vi "ChessTopVI.vi"() -> ()   [LabVIEW 2014]
panel:
  out "Whose Turn":string
  out "Draw":bool
  out "Black:":string
  out "Target Piece":i32
  out "Selected Piece":i32
  out "White:":string
  out "LastMovePiece":cluster{"Row":i32, "Column":i32, "IsMove":bool}
  out "AttachablePositionIndexes":i32[](array[numeric])
  out "AttachablePosition":bool[][](array[boolean])
  out "Target Piece Index":i32
  out "Selected Piece Index":i32
  in  "stop":bool
  out "Board":i32[][](array[numeric])=[[-3, -5, -4, -2, -1, -4, -5, -3], [-6, -6, -6, -6, -6, -6, -6, -6], [0, 0, 0, 0, 0, 0, 0, 0], [0, 0, 0, 0, 0, 0, 0, 0], [0, 0, 0, 0, 0, 0, 0, 0], [0, 0, 0, 0, 0, 0, 0, 0], [6, 6, 6, 6, 6, 6, 6, 6], [3, 5, 4, 2, 1, 4, 5, 3]]
  out "Black/White Turn (T/F)":bool
  out "Castling State":bool[][](array[boolean])
  in  "Cluster":T1
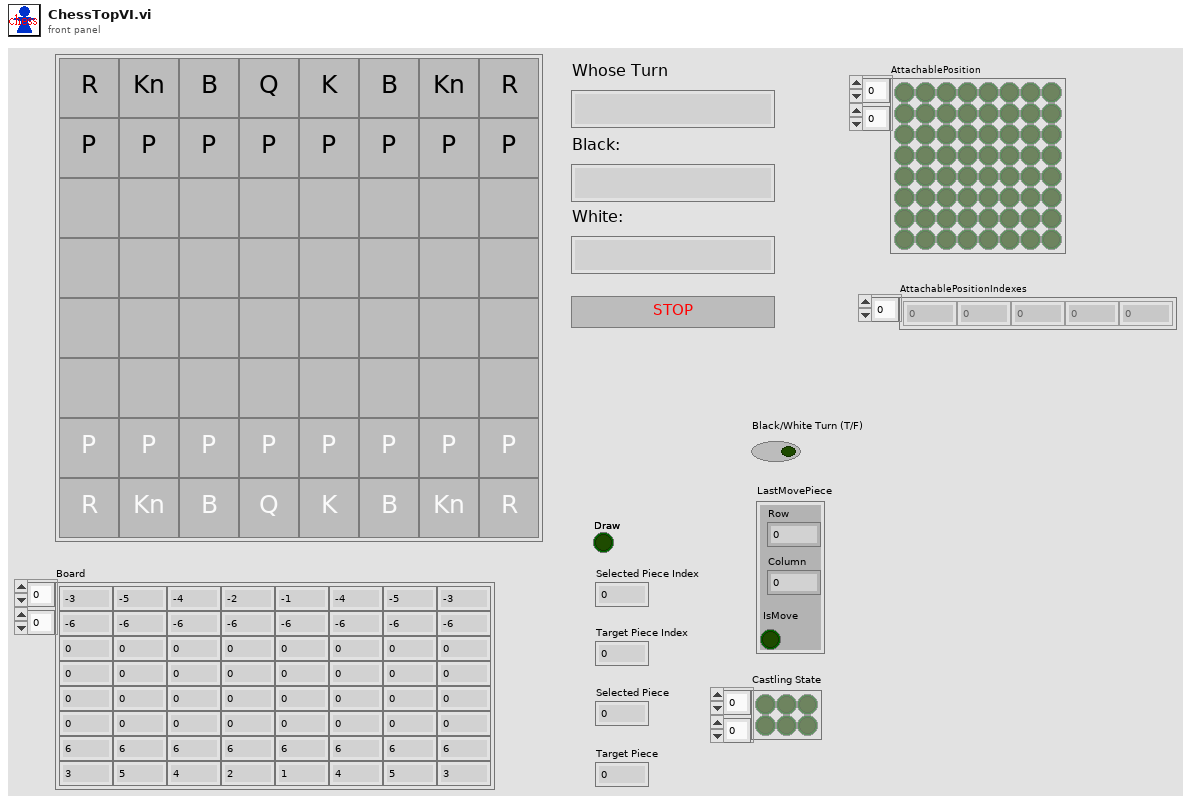
[diagram p1: front panel]
types:
  T1 = cluster{"OK Button":bool, "OK Button 2":bool, "OK Button 3":bool, "OK Button 4":bool, "OK Button 5":bool, "OK Button 6":bool, "OK Button 3":bool, "OK Button 7":bool, "OK Button 8":bool, "OK Button 9":bool, "OK Button 10":bool, "OK Button 11":bool, "OK Button 12":bool, "OK Button 13":bool, "OK Button 14":bool, "OK Button 15":bool, "OK Button 16":bool, "OK Button 17":bool, "OK Button 18":bool, "OK Button 19":bool, "OK Button 20":bool, "OK Button 21":bool, "OK Button 22":bool, "OK Button 23":bool, "OK Button 24":bool, "OK Button 25":bool, "OK Button 26":bool, "OK Button 27":bool, "OK Button 28":bool, "OK Button 29":bool, "OK Button 30":bool, "OK Button 31":bool, "OK Button 32":bool, "OK Button 33":bool, "OK Button 34":bool, "OK Button 35":bool, "OK Button 36":bool, "OK Button 37":bool, "OK Button 38":bool, "OK Button 39":bool, "OK Button 40":bool, "OK Button 41":bool, "OK Button 42":bool, "OK Button 43":bool, "OK Button 44":bool, "OK Button 45":bool, "OK Button 46":bool, "OK Button 47":bool, "OK Button 48":bool, "OK Button 49":bool, "OK Button 50":bool, "OK Button 51":bool, "OK Button 52":bool, "OK Button 53":bool, "OK Button 54":bool, "OK Button 55":bool, "OK Button 56":bool, "OK Button 57":bool, "OK Button 58":bool, "OK Button 59":bool, "OK Button 60":bool, "OK Button 61":bool, "OK Button 62":bool, "OK Button 63":bool}
  T2 = enum16{"init", "wait", "selected", "move/attack", "promotion", "checkmate"}
  T3 = cluster{"[0]":bool, "[1]":bool, "[2]":bool, "[3]":bool, "[4]":bool, "[5]":bool, "[6]":bool, "[7]":bool, "[8]":bool, "[9]":bool, "[10]":bool, "[11]":bool, "[12]":bool, "[13]":bool, "[14]":bool, "[15]":bool, "[16]":bool, "[17]":bool, "[18]":bool, "[19]":bool, "[20]":bool, "[21]":bool, "[22]":bool, "[23]":bool, "[24]":bool, "[25]":bool, "[26]":bool, "[27]":bool, "[28]":bool, "[29]":bool, "[30]":bool, "[31]":bool, "[32]":bool, "[33]":bool, "[34]":bool, "[35]":bool, "[36]":bool, "[37]":bool, "[38]":bool, "[39]":bool, "[40]":bool, "[41]":bool, "[42]":bool, "[43]":bool, "[44]":bool, "[45]":bool, "[46]":bool, "[47]":bool, "[48]":bool, "[49]":bool, "[50]":bool, "[51]":bool, "[52]":bool, "[53]":bool, "[54]":bool, "[55]":bool, "[56]":bool, "[57]":bool, "[58]":bool, "[59]":bool, "[60]":bool, "[61]":bool, "[62]":bool, "[63]":bool}
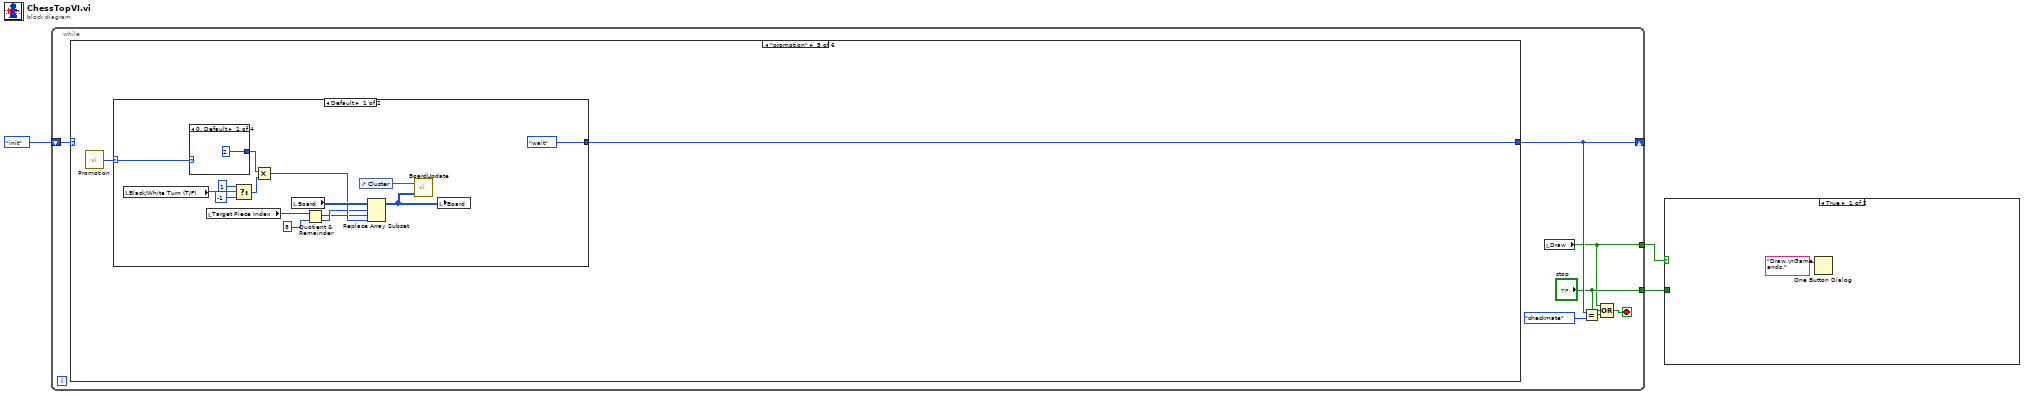
[diagram p0: block diagram]
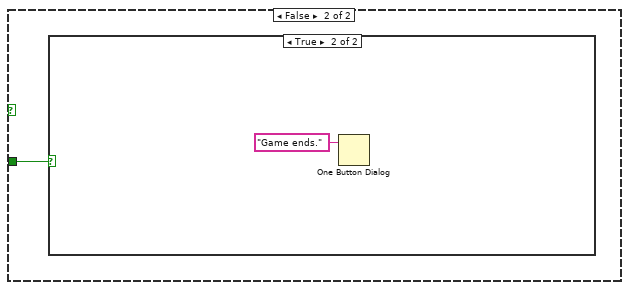
[diagram p2: hidden frame]
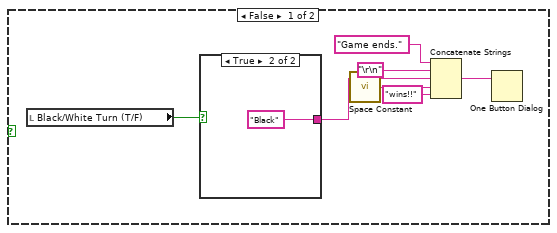
[diagram p3: hidden frame]
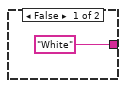
[diagram p4: hidden frame]
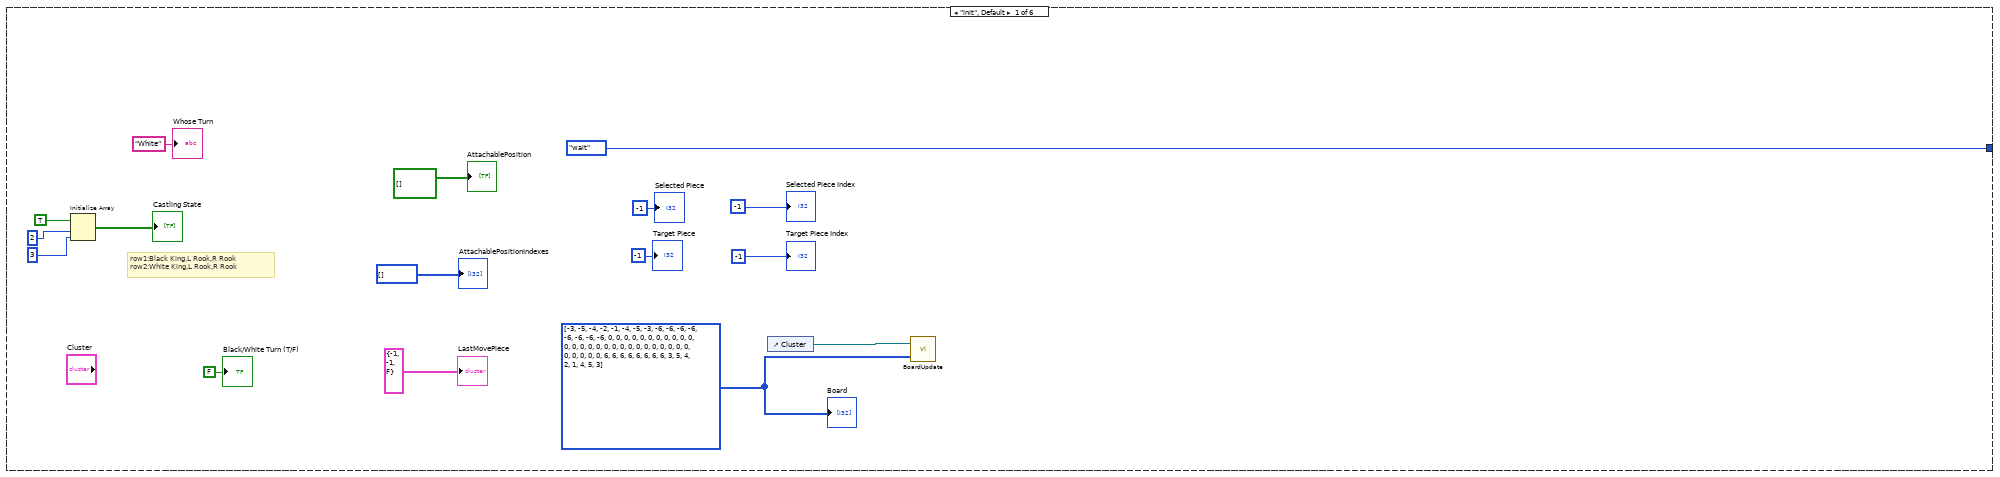
[diagram p5: hidden frame]
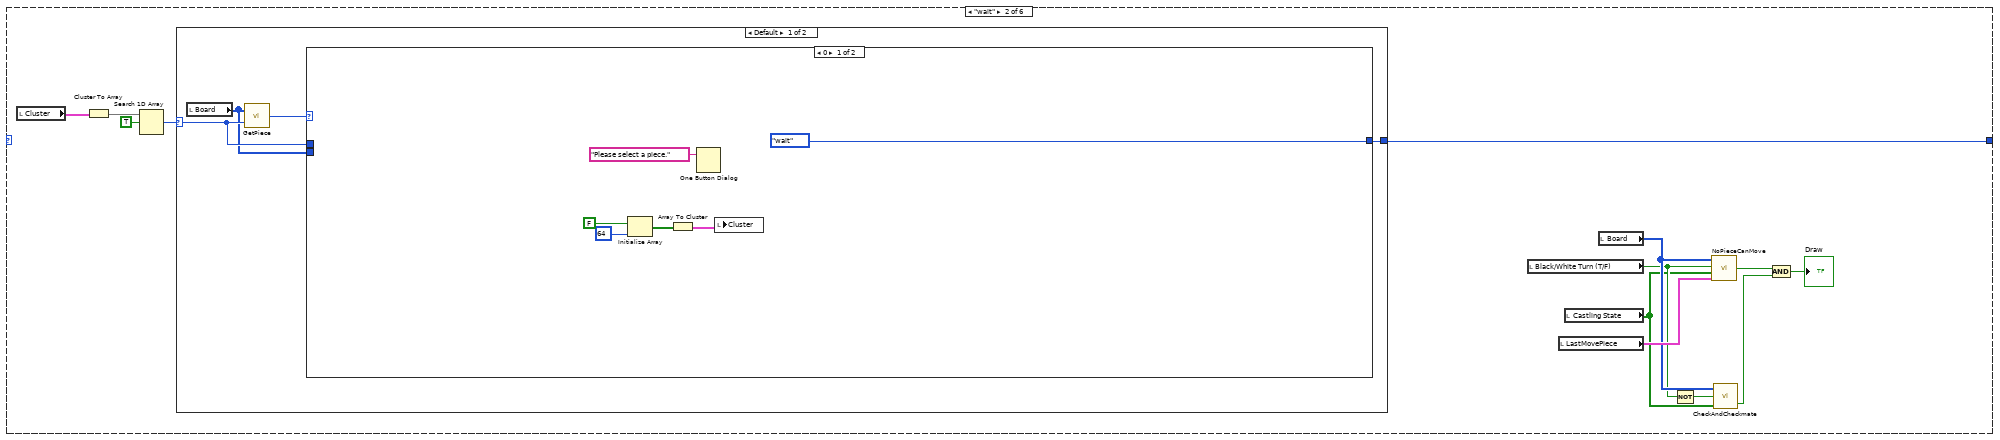
[diagram p6: hidden frame]
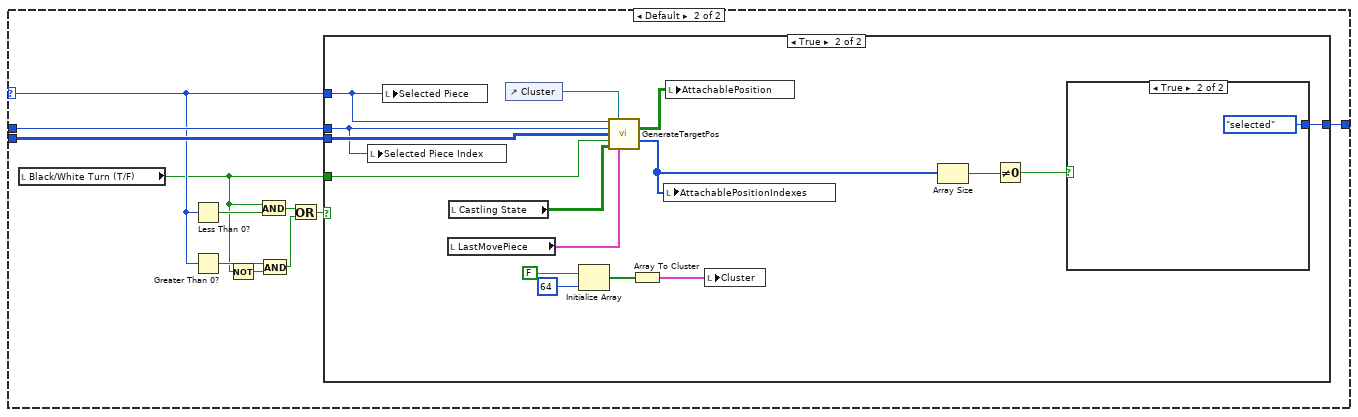
[diagram p7: hidden frame]
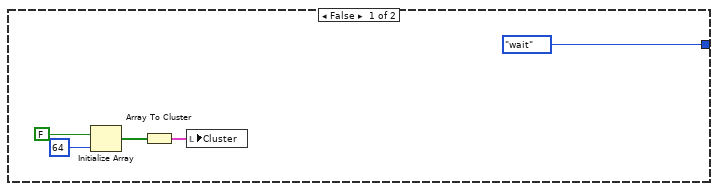
[diagram p8: hidden frame]
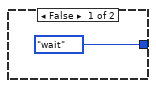
[diagram p9: hidden frame]
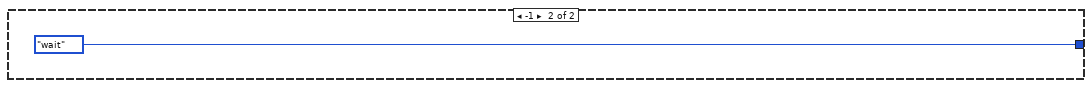
[diagram p10: hidden frame]
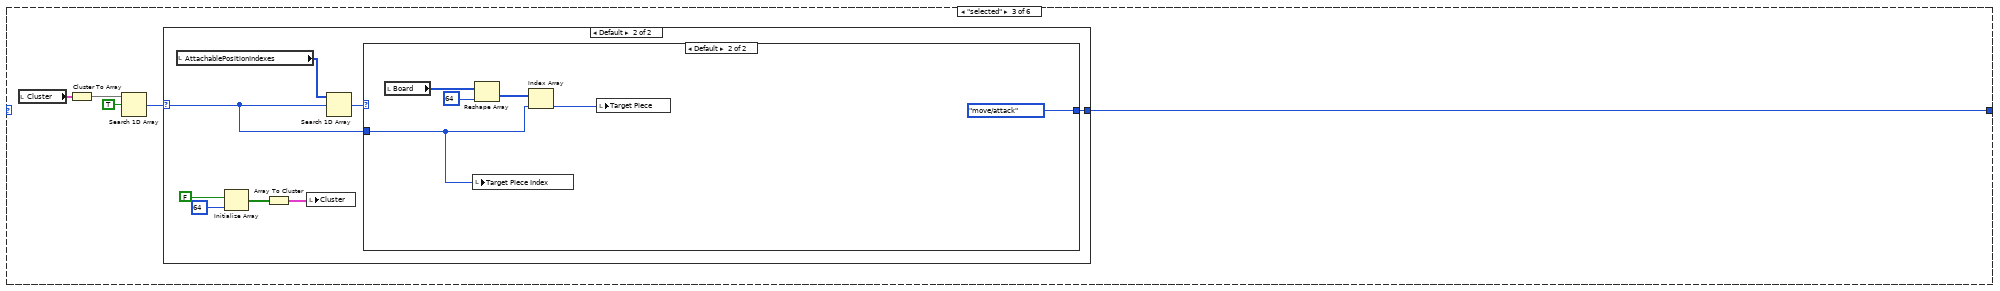
[diagram p11: hidden frame]
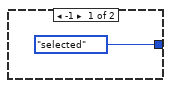
[diagram p12: hidden frame]
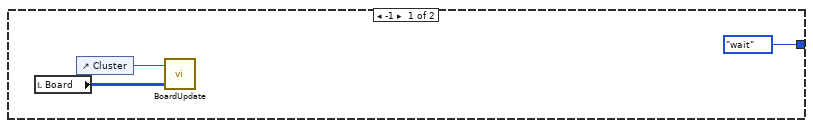
[diagram p13: hidden frame]
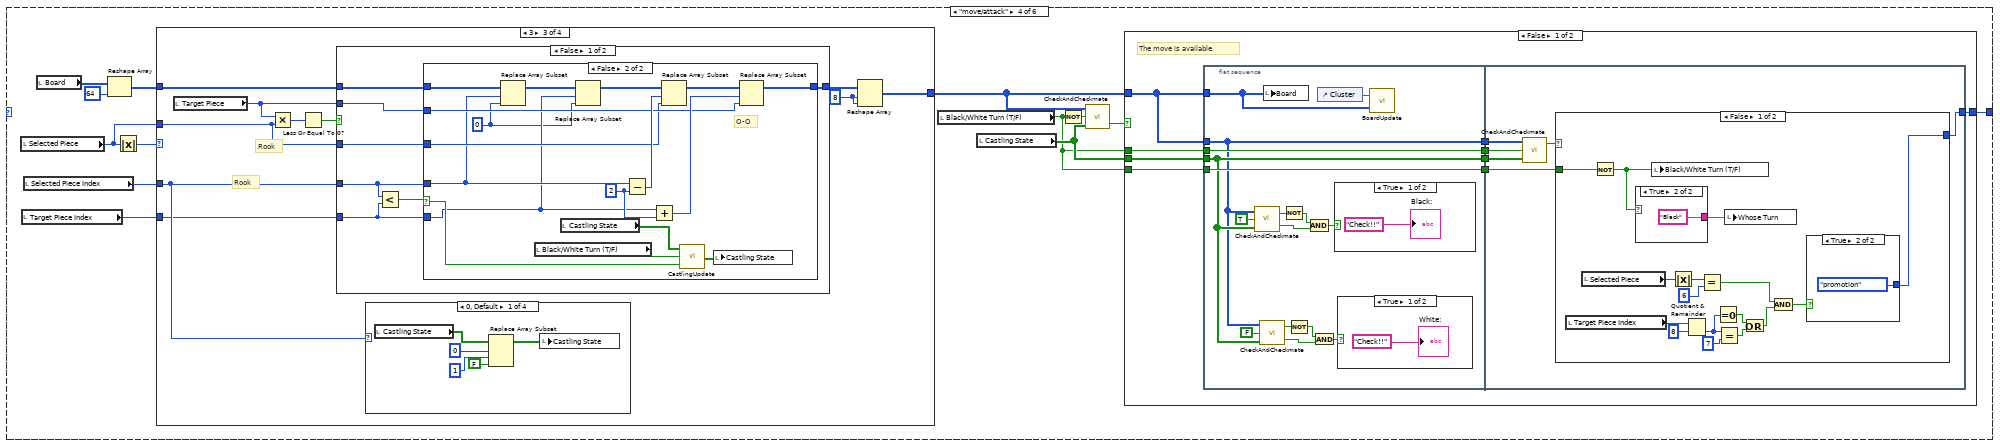
[diagram p14: hidden frame]
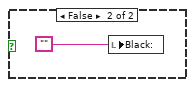
[diagram p15: hidden frame]
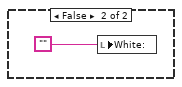
[diagram p16: hidden frame]
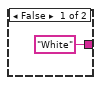
[diagram p17: hidden frame]
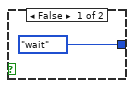
[diagram p18: hidden frame]
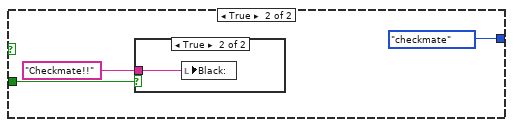
[diagram p19: hidden frame]
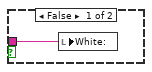
[diagram p20: hidden frame]
diagram:
  n1 = while {
    shift-right: [w8] -> _
    shift-left: T2."init" -> [w9]
    tunnel: ["stop"] -> w2
    tunnel: [w4] -> w1
    stop <- w6 stop-if-true
    n2 = case shown="\"promotion\"" w9 {
      tunnel: [T2."wait" w36 w89 w111 w412 T2."checkmate"] -> w8
      frame "init", Default {
        w12 = i32[][] [[-3, -5, -4, -2, -1, -4, -5, -3], [-6, -6, -6, -6, -6, -6, -6, -6], [0, 0, 0, 0, 0, 0, 0, 0], [0, 0, 0, 0, 0, 0, 0, 0], [0, 0, 0, 0, 0, 0, 0, 0], [0, 0, 0, 0, 0, 0, 0, 0], [6, 6, 6, 6, 6, 6, 6, 6], [3, 5, 4, 2, 1, 4, 5, 3]] ("Board")
        # "row1:Black King,L Rook,R Rook\nrow2:White King,L Rook,R Rook"
        n3 = Initialize Array(TRUE, 2, 3) -> (→"Castling State":bool[][])
        n4 = control-ref of="Cluster"() -> (w26:refnum<vi>)
        n5 = call "BoardUpdate.vi"("Array"=w12, "Clust Refnum"=w26) -> ()  [unwired: 1 in]
        "Black/White Turn (T/F)" <- FALSE ("Black/White Turn (T/F)")
        "Board" <- w12
        "LastMovePiece" <- cluster{"Row":i32, "Column":i32, "IsMove":bool} {"Row"=-1, "Column"=-1, "IsMove"=FALSE} ("LastMovePiece")
        "Selected Piece Index" <- -1 ("Selected Piece Index")
        "AttachablePosition" <- bool[][] [] ("AttachablePosition")
        "AttachablePositionIndexes" <- i32[] [] ("AttachablePositionIndexes")
        "Target Piece Index" <- -1 ("Target Index")
        "Selected Piece" <- -1 ("Selected Piece")
        "Target Piece" <- -1 ("Target Piece")
        "Whose Turn" <- "White" ("Whose Turn")
      }
      frame "wait" {
        n6 = local read "Cluster"() -> (w39:T1)
        n7 = Cluster To Array(cluster=w39) -> (array=w35:bool[])
        n8 = Search 1D Array(1D array=w35, element=TRUE) -> (index of element=w37:i32)  [unwired: 1 in]
        n9 = case shown="Default" w37 {
          selector: w37 -> [w41 _]
          tunnel: [w43 T2."wait"] -> w36
          frame Default {
            n10 = local read "Board"() -> (w40:i32[][])
            n11 = call "GetPiece.vi"("PieceIndex"=w41, "Board"=w40) -> ("Piece"=w42:i32)
            n12 = case shown="0" w42 {
              selector: w42 -> [_ w57]
              tunnel: [T2."wait" w60] -> w43
              tunnel: w41 -> [_ w58]
              tunnel: w40 -> [_ w59]
              frame 0 {
                n13 = Initialize Array(FALSE ("new element/subarray"), 64 ("dimension size")) -> (w47:bool[])
                n14 = Array To Cluster(array=w47) -> (cluster=w44:T3)
                n15 = One Button Dialog(message="Please select a piece.") -> ()  [unwired: 1 in, 1 out]
                n16 = local write "Cluster"(w44) -> ()
              }
              frame Default {
                n17 = local read "Black/White Turn (T/F)"() -> (w50:bool)
                n18 = Less Than 0?(x=w57) -> (x < 0?=w56:bool)
                n19 = Greater Than 0?(x=w57) -> (x > 0?=w53:bool)
                n20 = Not(x=w50) -> (.not. x?=w51:bool)
                n21 = And(x=w50, y=w56) -> (x .and. y?=w54:bool)
                n22 = And(x=w53, y=w51) -> (x .and. y?=w52:bool)
                n23 = Or(x=w54, y=w52) -> (x .or. y?=w55:bool)
                n24 = case shown="True" w55 {
                  tunnel: [T2."wait" w81] -> w60
                  tunnel: w59 -> [_ w78]
                  tunnel: w58 -> [_ w68]
                  tunnel: w57 -> [_ w67]
                  tunnel: w50 -> [_ w66]
                  frame False {
                    n25 = Initialize Array(FALSE ("new element/subarray"), 64 ("dimension size")) -> (w64:bool[])
                    n26 = Array To Cluster(array=w64) -> (cluster=w61:T3)
                    n27 = local write "Cluster"(w61) -> ()
                  }
                  frame True {
                    n28 = local write "Selected Piece Index"(w68) -> ()
                    n29 = local write "Selected Piece"(w67) -> ()
                    n30 = local read "LastMovePiece"() -> (w76:cluster{"Row":i32, "Column":i32, "IsMove":bool})
                    n31 = local read "Castling State"() -> (w77:bool[][])
                    n32 = control-ref of="Cluster"() -> (w79:refnum<vi>)
                    n33 = Initialize Array(FALSE ("new element/subarray"), 64 ("dimension size")) -> (w74:bool[])
                    n34 = call "GenerateTargetPos.vi"("Piece"=w67, "Clust Refnum"=w79, "Index"=w68, "Board"=w78, "Black/White Turn (T/F)"=w66, "Castling State"=w77, "LastMovePiece"=w76) -> ("AttachablePosition"=w80:bool[][], "AttachablePositionIndexes"=w71:i32[])  [unwired: 7 in]
                    n35 = Array To Cluster(array=w74) -> (cluster=w75:T3)
                    n36 = local write "AttachablePositionIndexes"(w71) -> ()
                    n37 = local write "AttachablePosition"(w80) -> ()
                    n38 = local write "Cluster"(w75) -> ()
                    n39 = Array Size(array=w71) -> (size(s)=w70:i32)
                    n40 = Not Equal To 0?(x=w70) -> (x != 0?=w69:bool)
                    n41 = case shown="True" w69 {
                      tunnel: [T2."wait" T2."selected"] -> w81
                      frame False {
                      }
                      frame True {
                      }
                    }
                  }
                }
              }
            }
          }
          frame -1 {
          }
        }
        n42 = local read "Black/White Turn (T/F)"() -> (w32:bool)
        n43 = local read "LastMovePiece"() -> (w34:cluster{"Row":i32, "Column":i32, "IsMove":bool})
        n44 = local read "Castling State"() -> (w31:bool[][])
        n45 = local read "Board"() -> (w33:i32[][])
        n46 = Not(x=w32) -> (.not. x?=w30:bool)
        n47 = call "NoPieceCanMove.vi"("LastMovePiece"=w34, "Castling State"=w31, "Black/White Turn (T/F)"=w32, "Board"=w33) -> ("NoPieceCanMove"=w28:bool)
        n48 = call "CheckAndCheckmate.vi"("Castling State"=w31, "Black/White Turn (T/F)"=w30, "Board"=w33) -> ("Check"=w29:bool)  [unwired: 1 out]
        n49 = And(x=w28, y=w29) -> (x .and. y?=→"Draw":bool)
      }
      frame "selected" {
        n50 = local read "Cluster"() -> (w86:T1)
        n51 = Cluster To Array(cluster=w86) -> (array=w87:bool[])
        n52 = Search 1D Array(1D array=w87, element=TRUE) -> (index of element=w85:i32)  [unwired: 1 in]
        n53 = case shown="Default" w85 {
          selector: w85 -> [_ w95]
          tunnel: [T2."selected" w98] -> w89
          frame -1 {
          }
          frame Default {
            n54 = local read "AttachablePositionIndexes"() -> (w97:i32[])
            n55 = Initialize Array(FALSE ("new element/subarray"), 64 ("dimension size")) -> (w91:bool[])
            n56 = Array To Cluster(array=w91) -> (cluster=w94:T3)
            n57 = local write "Cluster"(w94) -> ()
            n58 = Search 1D Array(1D array=w97, element=w95) -> (index of element=w96:i32)  [unwired: 1 in]
            n59 = case shown="Default" w96 {
              tunnel: [T2."wait" T2."move/attack"] -> w98
              tunnel: w95 -> [_ w103]
              frame -1 {
                n60 = local read "Board"() -> (w100:i32[][])
                n61 = control-ref of="Cluster"() -> (w99:refnum<vi>)
                n62 = call "BoardUpdate.vi"("Array"=w100, "Clust Refnum"=w99) -> ()  [unwired: 1 in]
              }
              frame Default {
                n63 = local read "Board"() -> (w106:i32[][])
                n64 = local write "Target Piece Index"(w103) -> ()
                n65 = Reshape Array(w106, 64 ("dimension size")) -> (w104:i32[])
                n66 = Index Array(array=w104, index=w103) -> (element=w102:i32)
                n67 = local write "Target Piece"(w102) -> ()
              }
            }
          }
        }
      }
      frame "move/attack" {
        n68 = local read "Selected Piece"() -> (w117:i32)
        n69 = local read "Target Piece Index"() -> (w118:i32)
        n70 = local read "Selected Piece Index"() -> (w119:i32)
        n71 = local read "Board"() -> (w115:i32[][])
        n72 = Reshape Array(w115, 64 ("dimension size")) -> (w114:i32[])
        n73 = Absolute Value(x=w117) -> (abs(x)=w120:i32)
        n74 = case shown="3" w120 {
          tunnel: w119 -> [w191 w200 w270 w349]
          tunnel: w118 -> [w186 w204 w269 w350]
          tunnel: w117 -> [w195 w198 w267 w347]
          tunnel: [w192 w202 w272 w346] -> w110
          tunnel: w114 -> [w190 w201 w274 w348]
          frame Default {
            w193 = 8 ("dimension size")
            n75 = Replace Array Subset(array=w190, new element=0 ("new element/subarray"), index=w191) -> (w196:i32[])
            n76 = Replace Array Subset(array=w196, new element=w195, index=w186) -> (w194:i32[])
            n77 = Reshape Array(w194, w193, w193) -> (w192:i32[][])
            n78 = Quotient & Remainder(x=w186, y=8) -> (x-y*floor(x/y)=w183:i32, floor(x/y)=w184:i32)
            n79 = local read "LastMovePiece"() -> (w188:cluster{"Row":i32, "Column":i32, "IsMove":bool})
            n80 = Bundle By Name(cluster=w188, "Row"=w184, "Column"=w183, "IsMove"=FALSE) -> (w187:cluster{"Row":i32, "Column":i32, "IsMove":bool})
            n81 = local write "LastMovePiece"(w187) -> ()
          }
          frame 1 {
            w205 = 8 ("dimension size")
            n82 = case shown="4, Default" w200 {
              frame 4, Default {
                n83 = local read "Castling State"() -> (w212:bool[][])
                n84 = Replace Array Subset(array=w212, new element=FALSE ("new element/subarray"), index (row)=0, index (col)=0 ("disabled index (col)")) -> (w208:bool[][])
                n85 = local write "Castling State"(w208) -> ()
              }
              frame 60 {
                n86 = local read "Castling State"() -> (w217:bool[][])
                n87 = Replace Array Subset(array=w217, new element=FALSE ("new element/subarray"), index (row)=1, index (col)=0 ("disabled index (col)")) -> (w213:bool[][])
                n88 = local write "Castling State"(w213) -> ()
              }
            }
            n89 = local read "Target Piece"() -> (w199:i32)
            n90 = Multiply(x=w199, y=w198) -> (x*y=w207:i32)
            n91 = Less Or Equal To 0?(x=w207) -> (x <= 0?=w206:bool)
            n92 = case shown="False" w206 {
              tunnel: w201 -> [w221 w264]
              tunnel: w200 -> [w222 w263]
              tunnel: w204 -> [w223 w262]
              tunnel: w198 -> [w219 w261]
              tunnel: [w220 w260] -> w203
              tunnel: w199 -> [w218 _]
              frame False {
                n93 = Greater?(x=w222, y=w223) -> (0:w224:bool)
                n94 = case shown="True" w224 {
                  selector: w224 -> [w232 w250]
                  tunnel: w223 -> [w226 w244]
                  tunnel: w222 -> [w227 w245]
                  tunnel: w221 -> [w240 w259]
                  tunnel: [w238 w257] -> w220
                  tunnel: w219 -> [w231 w249]
                  tunnel: w218 -> [w230 w248]
                  frame True {
                    w225 = 0
                    # "O-O-O"
                    n95 = Replace Array Subset(array=w240, new element=w225, index=w227) -> (w229:i32[])
                    n96 = local read "Black/White Turn (T/F)"() -> (w235:bool)
                    n97 = local read "Castling State"() -> (w234:bool[][])
                    n98 = Replace Array Subset(array=w229, new element=w225, index=w226) -> (w228:i32[])
                    n99 = Subtract(x=w227, y=2) -> (x-y=w237:i32)
                    n100 = Add(x=3, y=w226) -> (x+y=w236:i32)
                    n101 = call "CastlingUpdate.vi"("L/R (T/F)"=w232, "Black/White Turn (T/F)"=w235, "Castling State"=w234) -> ("Update Castling State"=w233:bool[][])
                    n102 = Replace Array Subset(array=w228, new element=w231, index=w237) -> (w239:i32[])
                    n103 = local write "Castling State"(w233) -> ()
                    n104 = Replace Array Subset(array=w239, new element=w230, index=w236) -> (w238:i32[])
                  }
                  frame False {
                    w243 = 0
                    w254 = 2 ("y")
                    # "O-O"
                    n105 = Replace Array Subset(array=w259, new element=w243, index=w245) -> (w247:i32[])
                    n106 = local read "Black/White Turn (T/F)"() -> (w253:bool)
                    n107 = local read "Castling State"() -> (w252:bool[][])
                    n108 = Replace Array Subset(array=w247, new element=w243, index=w244) -> (w246:i32[])
                    n109 = Add(x=w245, y=w254) -> (x+y=w256:i32)
                    n110 = Subtract(x=w244, y=w254) -> (x-y=w255:i32)
                    n111 = call "CastlingUpdate.vi"("L/R (T/F)"=w250, "Black/White Turn (T/F)"=w253, "Castling State"=w252) -> ("Update Castling State"=w251:bool[][])
                    n112 = Replace Array Subset(array=w246, new element=w249, index=w256) -> (w258:i32[])
                    n113 = local write "Castling State"(w251) -> ()
                    n114 = Replace Array Subset(array=w258, new element=w248, index=w255) -> (w257:i32[])
                  }
                }
              }
              frame True {
                # "attack/move"
                n115 = Replace Array Subset(array=w264, new element=0 ("new element/subarray"), index=w263) -> (w265:i32[])
                n116 = Replace Array Subset(array=w265, new element=w261, index=w262) -> (w260:i32[])
              }
            }
            n117 = Reshape Array(w203, w205, w205) -> (w202:i32[][])
          }
          frame 3 {
            w273 = 8 ("dimension size")
            # "Rook"
            # "Rook"
            n118 = local read "Target Piece"() -> (w268:i32)
            n119 = Multiply(x=w268, y=w267) -> (x*y=w276:i32)
            n120 = Less Or Equal To 0?(x=w276) -> (x <= 0?=w275:bool)
            n121 = case shown="False" w275 {
              tunnel: w274 -> [w282 w323]
              tunnel: [w283 w322] -> w271
              tunnel: w270 -> [w279 w321]
              tunnel: w269 -> [w280 w320]
              tunnel: w267 -> [w277 w319]
              tunnel: w268 -> [w278 _]
              frame False {
                n122 = Less?(x=w279, y=w280) -> (x < y?=w281:bool)
                n123 = case shown="False" w281 {
                  selector: w281 -> [w289 w310]
                  tunnel: w280 -> [w285 w303]
                  tunnel: w279 -> [w286 w304]
                  tunnel: w282 -> [w300 w318]
                  tunnel: [w298 w316] -> w283
                  tunnel: w277 -> [w293 w311]
                  tunnel: w278 -> [w294 w312]
                  frame True {
                    w284 = 0 ("Target Piece")
                    # "O-O-O"
                    n124 = Replace Array Subset(array=w300, new element=w284, index=w286) -> (w288:i32[])
                    n125 = local read "Black/White Turn (T/F)"() -> (w292:bool)
                    n126 = Replace Array Subset(array=w288, new element=w284, index=w285) -> (w287:i32[])
                    n127 = local read "Castling State"() -> (w291:bool[][])
                    n128 = Add(x=w286, y=3) -> (x+y=w297:i32)
                    n129 = Subtract(x=w285, y=2 ("x")) -> (x-y=w296:i32)
                    n130 = Replace Array Subset(array=w287, new element=w293, index=w297) -> (w299:i32[])
                    n131 = call "CastlingUpdate.vi"("L/R (T/F)"=w289, "Black/White Turn (T/F)"=w292, "Castling State"=w291) -> ("Update Castling State"=w290:bool[][])
                    n132 = local write "Castling State"(w290) -> ()
                    n133 = Replace Array Subset(array=w299, new element=w294, index=w296) -> (w298:i32[])
                  }
                  frame False {
                    w302 = 0 ("new element/subarray")
                    w313 = 2 ("y")
                    # "O-O"
                    n134 = Replace Array Subset(array=w318, new element=w302, index=w304) -> (w306:i32[])
                    n135 = local read "Black/White Turn (T/F)"() -> (w307:bool)
                    n136 = local read "Castling State"() -> (w308:bool[][])
                    n137 = Replace Array Subset(array=w306, new element=w302, index=w303) -> (w305:i32[])
                    n138 = Subtract(x=w304, y=w313) -> (x-y=w315:i32)
                    n139 = Add(x=w303, y=w313) -> (x+y=w314:i32)
                    n140 = Replace Array Subset(array=w305, new element=w311, index=w315) -> (w317:i32[])
                    n141 = call "CastlingUpdate.vi"("L/R (T/F)"=w310, "Black/White Turn (T/F)"=w307, "Castling State"=w308) -> ("Update Castling State"=w309:bool[][])
                    n142 = local write "Castling State"(w309) -> ()
                    n143 = Replace Array Subset(array=w317, new element=w312, index=w314) -> (w316:i32[])
                  }
                }
              }
              frame True {
                # "attack/move"
                n144 = Replace Array Subset(array=w323, new element=0 ("new element/subarray"), index=w321) -> (w324:i32[])
                n145 = Replace Array Subset(array=w324, new element=w319, index=w320) -> (w322:i32[])
              }
            }
            n146 = case shown="0, Default" w270 {
              frame 0, Default {
                n147 = local read "Castling State"() -> (w330:bool[][])
                n148 = Replace Array Subset(array=w330, new element=FALSE ("new element/subarray"), index (row)=0, index (col)=1 ("disabled index (col)")) -> (w326:bool[][])
                n149 = local write "Castling State"(w326) -> ()
              }
              frame 7 {
                n150 = local read "Castling State"() -> (w335:bool[][])
                n151 = Replace Array Subset(array=w335, new element=FALSE ("new element/subarray"), index (row)=0, index (col)=2 ("disabled index (col)")) -> (w331:bool[][])
                n152 = local write "Castling State"(w331) -> ()
              }
              frame 56 {
                n153 = local read "Castling State"() -> (w340:bool[][])
                n154 = Replace Array Subset(array=w340, new element=FALSE ("new element/subarray"), index (row)=1, index (col)=1 ("disabled index (col)")) -> (w336:bool[][])
                n155 = local write "Castling State"(w336) -> ()
              }
              frame 63 {
                n156 = local read "Castling State"() -> (w345:bool[][])
                n157 = Replace Array Subset(array=w345, new element=FALSE ("new element/subarray"), index (row)=1, index (col)=2 ("disabled index (col)")) -> (w341:bool[][])
                n158 = local write "Castling State"(w341) -> ()
              }
            }
            n159 = Reshape Array(w271, w273, w273) -> (w272:i32[][])
          }
          frame 6 {
            n160 = Subtract(x=w349, y=w350) -> (x-y=w352:i32)
            n161 = Absolute Value(x=w352) -> (abs(x)=w351:i32)
            n162 = case shown="Default" w351 {
              tunnel: w350 -> [w371 w398]
              tunnel: w349 -> [w372 w409]
              tunnel: w348 -> [w368 w410]
              tunnel: w347 -> [w360 w403]
              tunnel: [w365 w405] -> w346
              frame Default {
                w369 = 8 ("dimension size")
                w370 = 8
                # "attack: different column"
                n163 = local read "LastMovePiece"() -> (w356:cluster{"Row":i32, "Column":i32, "IsMove":bool})
                n164 = Quotient & Remainder(x=w372, y=w370) -> (x-y*floor(x/y)=w358:i32, floor(x/y)=w359:i32)
                n165 = Quotient & Remainder(x=w371, y=w370) -> (x-y*floor(x/y)=w362:i32, floor(x/y)=w361:i32)
                n166 = Reshape Array(w368, w369, w369) -> (w366:i32[][])
                n167 = Unbundle By Name(w356) -> ("Row"=w364:i32, "Column"=w363:i32, "IsMove"=w367:bool)
                n168 = case shown="False" w367 {
                  tunnel: w366 -> [w382 w395]
                  tunnel: [w380 w393] -> w365
                  tunnel: w364 -> [_ w392]
                  tunnel: w363 -> [_ w391]
                  tunnel: w362 -> [w375 w384]
                  tunnel: w361 -> [w374 w385]
                  tunnel: w360 -> [w379 w390]
                  tunnel: w359 -> [w377 w388]
                  tunnel: w358 -> [w378 w387]
                  tunnel: [w374 w385] -> w355
                  tunnel: [w375 w384] -> w354
                  tunnel: [FALSE FALSE] -> w353
                  frame False {
                    n169 = Replace Array Subset(array=w382, new element=0 ("new element/subarray"), index (row)=w377, index (col)=w378) -> (w381:i32[][])
                    n170 = Replace Array Subset(array=w381, new element=w379, index (row)=w374, index (col)=w375) -> (w380:i32[][])
                  }
                  frame True {
                    w386 = 0 ("new element/subarray")
                    # "En passant:吃過路兵"
                    n171 = Replace Array Subset(array=w395, new element=w386, index (row)=w388, index (col)=w387) -> (w389:i32[][])
                    n172 = Replace Array Subset(array=w389, new element=w386, index (row)=w392, index (col)=w391) -> (w394:i32[][])
                    n173 = Replace Array Subset(array=w394, new element=w390, index (row)=w385, index (col)=w384) -> (w393:i32[][])
                  }
                }
                n174 = Bundle By Name(cluster=w356, "Row"=w355, "Column"=w354, "IsMove"=w353) -> (w357:cluster{"Row":i32, "Column":i32, "IsMove":bool})
                n175 = local write "LastMovePiece"(w357) -> ()
              }
              frame 8, 16 {
                w404 = 8 ("dimension size")
                # "move: same column"
                n176 = Replace Array Subset(array=w410, new element=0 ("new element/subarray"), index=w409) -> (w407:i32[])
                n177 = Replace Array Subset(array=w407, new element=w403, index=w398) -> (w406:i32[])
                n178 = Quotient & Remainder(x=w398, y=8) -> (x-y*floor(x/y)=w399:i32, floor(x/y)=w400:i32)
                n179 = local read "LastMovePiece"() -> (w401:cluster{"Row":i32, "Column":i32, "IsMove":bool})
                n180 = Reshape Array(w406, w404, w404) -> (w405:i32[][])
                n181 = Bundle By Name(cluster=w401, "Row"=w400, "Column"=w399, "IsMove"=TRUE) -> (w402:cluster{"Row":i32, "Column":i32, "IsMove":bool})
                n182 = local write "LastMovePiece"(w402) -> ()
              }
            }
          }
        }
        n183 = local read "Black/White Turn (T/F)"() -> (w108:bool)
        n184 = local read "Castling State"() -> (w109:bool[][])
        n185 = Not(x=w108) -> (.not. x?=w113:bool)
        n186 = call "CheckAndCheckmate.vi"("Castling State"=w109, "Black/White Turn (T/F)"=w113, "Board"=w110) -> ("Check"=w112:bool)  [unwired: 1 out]
        n187 = case shown="False" w112 {
          tunnel: [w126 T2."selected"] -> w111
          tunnel: w110 -> [w121 _]
          tunnel: w108 -> [w129 _]
          tunnel: w109 -> [w128 _]
          tunnel: w108 -> [w127 _]
          frame False {
            # "The move is available."
            n188 = flat-sequence {
              tunnel: w121 -> [w130]
              tunnel: w127 -> [w144]
              tunnel: w128 -> [w131]
              tunnel: w129 -> [w145]
              tunnel: [w145] -> w125
              tunnel: [w131] -> w124
              tunnel: [w144] -> w123
              tunnel: [w130] -> w122
              tunnel: w121 -> [w142]
              tunnel: [w150] -> w126
              tunnel: w125 -> [w155]
              tunnel: w124 -> [w154]
              tunnel: w123 -> [w153]
              tunnel: w122 -> [w152]
              frame #0 {
                n189 = call "CheckAndCheckmate.vi"("Castling State"=w131, "Black/White Turn (T/F)"=TRUE, "Board"=w130) -> ("Check"=w135:bool, "Checkmate"=w137:bool)
                n190 = call "CheckAndCheckmate.vi"("Castling State"=w131, "Black/White Turn (T/F)"=FALSE, "Board"=w130) -> ("Check"=w138:bool, "Checkmate"=w141:bool)
                n191 = local write "Board"(w142) -> ()
                n192 = Not(x=w137) -> (.not. x?=w136:bool)
                n193 = Not(x=w141) -> (.not. x?=w139:bool)
                n194 = And(x=w136, y=w135) -> (x .and. y?=w134:bool)
                n195 = And(x=w139, y=w138) -> (x .and. y?=w140:bool)
                n196 = control-ref of="Cluster"() -> (w143:refnum<vi>)
                n197 = case shown="True" w134 {
                  frame True {
                    "Black:" <- "Check!!"
                  }
                  frame False {
                    n198 = local write "Black:"("") -> ()
                  }
                }
                n199 = case shown="True" w140 {
                  frame True {
                    "White:" <- "Check!!"
                  }
                  frame False {
                    n200 = local write "White:"("") -> ()
                  }
                }
                n201 = call "BoardUpdate.vi"("Array"=w142, "Clust Refnum"=w143) -> ()  [unwired: 1 in]
              }
              frame #1 {
                n202 = call "CheckAndCheckmate.vi"("Castling State"=w154, "Black/White Turn (T/F)"=w153, "Board"=w152) -> ("Checkmate"=w151:bool)  [unwired: 1 out]
                n203 = case shown="False" w151 {
                  tunnel: [w158 T2."checkmate"] -> w150
                  tunnel: w155 -> [w171 w176]
                  frame False {
                    n204 = local read "Target Piece Index"() -> (w167:i32)
                    n205 = local read "Selected Piece"() -> (w170:i32)
                    n206 = Not(x=w171) -> (.not. x?=w157:bool)
                    n207 = case shown="True" w157 {
                      tunnel: ["White" "Black"] -> w156
                      frame False {
                      }
                      frame True {
                      }
                    }
                    n208 = local write "Black/White Turn (T/F)"(w157) -> ()
                    n209 = Absolute Value(x=w170) -> (abs(x)=w169:i32)
                    n210 = Quotient & Remainder(x=w167, y=8) -> (floor(x/y)=w165:i32)  [unwired: 1 out]
                    n211 = Equal?(x=w169, y=6) -> (x = y?=w160:bool)
                    n212 = Equal To 0?(x=w165) -> (x = 0?=w162:bool)
                    n213 = Equal?(x=w165, y=7) -> (x = y?=w163:bool)
                    n214 = local write "Whose Turn"(w156) -> ()
                    n215 = Or(x=w162, y=w163) -> (x .or. y?=w161:bool)
                    n216 = And(x=w160, y=w161) -> (x .and. y?=w159:bool)
                    n217 = case shown="True" w159 {
                      tunnel: [T2."wait" T2."promotion"] -> w158
                      frame False {
                      }
                      frame True {
                      }
                    }
                  }
                  frame True {
                    n218 = case shown="True" w176 {
                      tunnel: "Checkmate!!" -> [w179 w180]
                      frame False {
                        n219 = local write "White:"(w179) -> ()
                      }
                      frame True {
                        n220 = local write "Black:"(w180) -> ()
                      }
                    }
                  }
                }
              }
            }
          }
          frame True {
            # "The move is not available."
            n221 = One Button Dialog(message="The move will make you be checked.") -> ()  [unwired: 1 in, 1 out]
          }
        }
      }
      frame "promotion" {
        n222 = call "Promotion.vi"() -> ("index of element"=w411:i32)  [unwired: 1 in]
        n223 = case shown="Default" w411 {
          selector: w411 -> [w427 _]
          tunnel: [T2."wait" T2."promotion"] -> w412
          frame Default {
            n224 = local read "Black/White Turn (T/F)"() -> (w414:bool)
            n225 = case shown="0, Default" w427 {
              tunnel: [2 3 4 5] -> w422
              frame 0, Default {
              }
              frame 1 {
              }
              frame 2 {
              }
              frame 3 {
              }
            }
            n226 = local read "Target Piece Index"() -> (w419:i32)
            n227 = Select(t=1, s=w414, f=-1) -> (s? t:f=w423:i32)
            n228 = Multiply(x=w422, y=w423) -> (x*y=w420:i32)
            n229 = local read "Board"() -> (w421:i32[][])
            n230 = Quotient & Remainder(x=w419, y=8) -> (x-y*floor(x/y)=w416:i32, floor(x/y)=w417:i32)
            n231 = control-ref of="Cluster"() -> (w415:refnum<vi>)
            n232 = Replace Array Subset(array=w421, new element=w420, index (row)=w417, index (col)=w416) -> (w413:i32[][])
            n233 = call "BoardUpdate.vi"("Array"=w413, "Clust Refnum"=w415) -> ()  [unwired: 1 in]
            n234 = local write "Board"(w413) -> ()
          }
          frame -1 {
          }
        }
      }
      frame "checkmate" {
        n235 = local read "Black/White Turn (T/F)"() -> (w436:bool)
        n236 = case shown="True" w436 {
          tunnel: ["White" "Black"] -> w435
          frame False {
          }
          frame True {
          }
        }
        n237 = Concatenate Strings(w435, " wins!!" ("string")) -> (w433:string)
        n238 = One Button Dialog(message=w433) -> ()  [unwired: 1 in, 1 out]
      }
    }
    n239 = local read "Draw"() -> (w4:bool)
    n240 = Equal?(x=w8, y=T2."checkmate") -> (x = y?=w7:bool)
    n241 = Compound Arithmetic op=OR(w4, "stop", w7) -> (w6:bool)
  }
  n242 = case shown="True" w1 {
    tunnel: w2 -> [_ w441]
    frame True {
      n243 = One Button Dialog(message="Draw.\nGame ends.") -> ()  [unwired: 1 in, 1 out]
    }
    frame False {
      n244 = case shown="True" w441 {
        frame False {
          n245 = local read "Black/White Turn (T/F)"() -> (w448:bool)
          n246 = case shown="True" w448 {
            tunnel: ["White" "Black"] -> w445
            frame False {
            }
            frame True {
            }
          }
          n247 = call <vilib>:"Space Constant.vi"() -> ("String"=w444:string)
          n248 = Concatenate Strings("Game ends." ("string"), "\r\n", w445, w444, "wins!!" ("string")) -> (w442:string)
          n249 = One Button Dialog(message=w442) -> ()  [unwired: 1 in, 1 out]
        }
        frame True {
          n250 = One Button Dialog(message="Game ends.") -> ()  [unwired: 1 in, 1 out]
        }
      }
    }
  }
